vi "CLD 11 Producer consumer events front panel.vi"() -> ()   [LabVIEW 2009]
doc: "CLD-Übung 11"
panel:
  out "Aktuelle Zielzeit":dbl
  out "Schritt 3":bool
  out "Schritt 2":bool
  out "Schritt 1":bool
  out "Zeit ist verstrichen":bool
  out "Verstrichene Zeit":string
  in  "Autom. zurücksetzen":bool
  in  "Zurücksetzen-Schaltfläche":bool
  in  "VI anhalten":bool
  in  "Zielzeit (s)":dbl
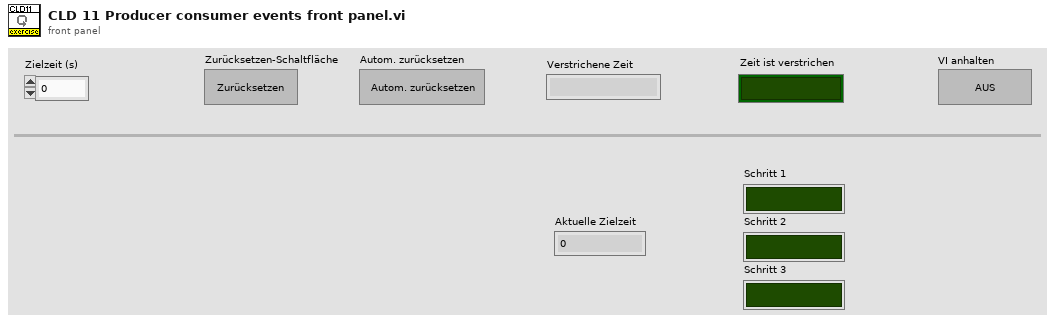
[diagram p1: front panel]
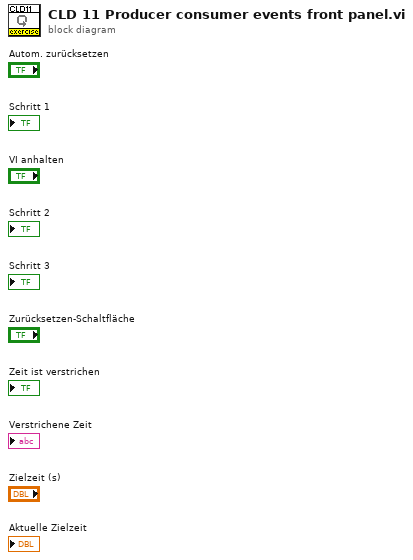
[diagram p0: block diagram]
diagram:
